vi "new_show_outside.vi"(10 "Multicolumn Listbox 2":refnum<vi>, 11 "Array":T1(array[cluster])) -> (0 "max value":i32)   [LabVIEW 2014]
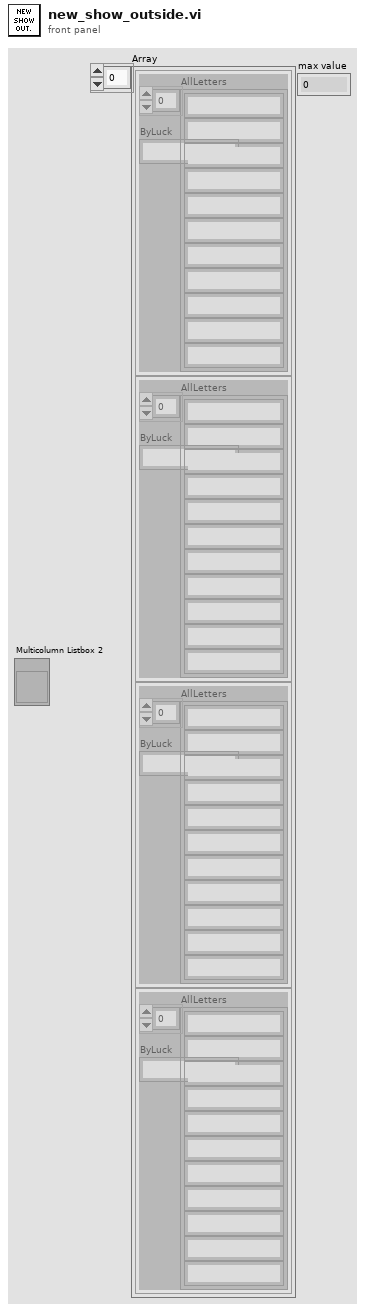
[diagram p1: front panel]
types:
  T1 = cluster{"AllLetters":string[], "ByLuck":string}[]
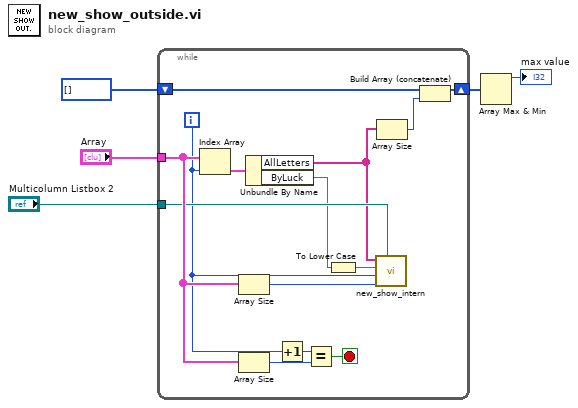
[diagram p0: block diagram]
diagram:
  n1 = while {
    tunnel: "Multicolumn Listbox 2" -> [w16]
    tunnel: "Array" -> [w18]
    shift-right: [w7] -> w2
    shift-left: i32[] [] -> [w6]
    i -> [w10]
    stop <- w19 stop-if-true
    n2 = Index Array(array=w18, index=w10) -> (element=w14:cluster{"AllLetters":string[], "ByLuck":string})
    n3 = Array Size(array=w18) -> (size(s)=w17:i32)
    n4 = Array Size(array=w18) -> (size(s)=w11:i32)
    n5 = Unbundle By Name(w14) -> ("AllLetters"=w9:string[], "ByLuck"=w13:string)
    n6 = Increment(x=w10) -> (x+1=w15:i32)
    n7 = Equal?(x=w15, y=w11) -> (x = y?=w19:bool)
    n8 = To Lower Case(string=w13) -> (all lower case string=w12:string)
    n9 = call "new_show_intern.vi"("reference"=w16, "lines"=w17, "x"=w10, "first letter to find"=w12, "Array"=w9) -> ()  [unwired: 7 in]
    n10 = Array Size(array=w9) -> (size(s)=w8:i32)
    n11 = Build Array (concatenate)(w6, w8) -> (w7:i32[])
  }
  n12 = Array Max & Min(array=w2) -> (max value=→"max value":i32)  [unwired: 3 out]
